vi "Read QD Settings.vi"(8 "error in (no error)":errorcluster, 11 "Dot Settings in":refnum<class "Dot Settings.lvclass">) -> (0 "error out":errorcluster, 2 "QD Settings":T1, 3 "Dot Settings out":refnum<class "Dot Settings.lvclass">)   [LabVIEW 2019, in "Dot Settings.lvclass"]
uses:
  Dot Settings.lvclass
  8c1048c6-e701-4974-b58d-e95050acfb0b.vi
  TypeDefs/QD Settings.ctl
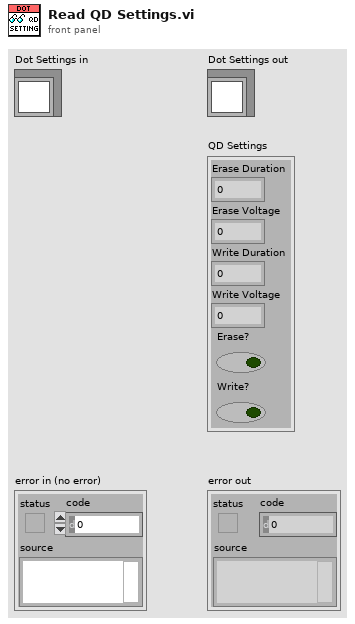
[diagram p1: front panel]
types:
  T1 = typedef "Dot Settings.lvclass/QD Settings.ctl" = cluster{"Erase Duration":dbl, "Erase Voltage":dbl, "Write Duration":dbl, "Write Voltage":dbl, "Erase?":bool, "Write?":bool}
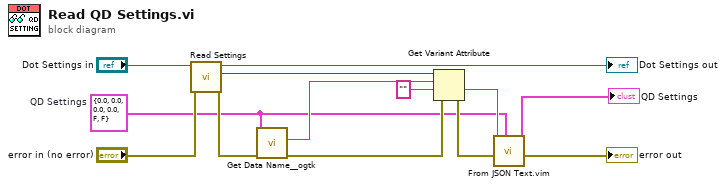
[diagram p0: block diagram]
diagram:
  w2 = T1 {"Erase Duration"=0.0, "Erase Voltage"=0.0, "Write Duration"=0.0, "Write Voltage"=0.0, "Erase?"=FALSE, "Write?"=FALSE}  # QD Settings
  n1 = call "Read Settings.vi"("error in (no error)"="error in (no error)", "Dot Settings in"="Dot Settings in") -> ("error out"=w7:errorcluster, "Settings"=w11:variant, "Dot Settings out"=→"Dot Settings out":refnum<class "Dot Settings.lvclass">)  [unwired: 7 in]
  n2 = call <userlib>:"Get Data Name__ogtk.vi"("error in (no error)"=w7, "Data"=w2) -> ("error out"=w9:errorcluster, "Data Name"=w10:string)  [unwired: 7 in, 1 out]
  n3 = Get Variant Attribute(Variant=w11, name=w10, default value (empty Variant)="", error in=w9) -> (value=w3:string, error out=w5:errorcluster)  [unwired: 2 out]
  n4 = call "From JSON Text.vim"("Data Type and Default Value"=w2, "error in (no error)"=w5, "JSON"=w3) -> ("error out"=→"error out":errorcluster, "Data out"=→"QD Settings":T1)  [unwired: 7 in]
